vi "Movimiento_2Ejes(SubVi).vi"(2 "Cluster":T1={"Dif_1"=0.0, "Dif_2"=0.0, "Motion Resource 2"="Eje Y", "Motion Resource 1"="Eje X", "Velocidad"=0.0, "Posición_1"=0.0, "Posición_2"=0.0}) -> (0 "Done":bool)   [LabVIEW 2017]
uses:
  <vilib>/Motion/Express/_s/nimc.fb.straightLineMove.startStraightLineMove.axis.modeAbsolute.0.vi
  <vilib>/Motion/BlockNode/FB.NIMotion.xnode
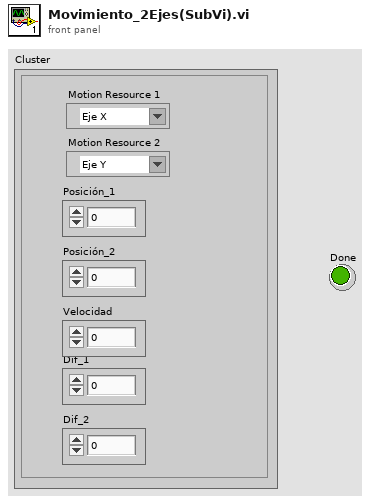
[diagram p1: front panel]
types:
  T1 = cluster{"Dif_1":dbl, "Dif_2":dbl, "Motion Resource 2":refnum<k21>, "Motion Resource 1":refnum<k21>, "Velocidad":dbl, "Posición_1":dbl, "Posición_2":dbl}
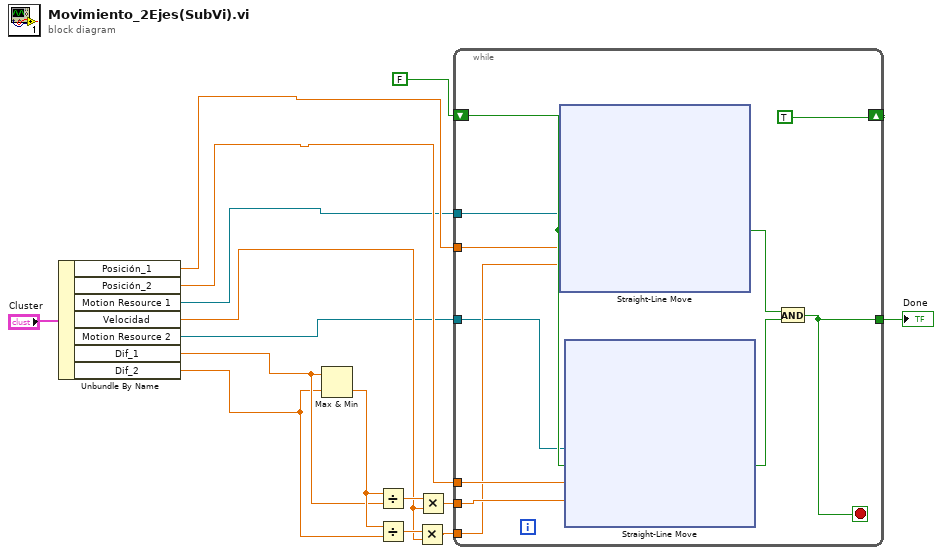
[diagram p0: block diagram]
diagram:
  n1 = Unbundle By Name("Cluster") -> ("Posición_1"=w7:dbl, "Posición_2"=w6:dbl, "Motion Resource 1"=w5:refnum<k21>, "Velocidad"=w4:dbl, "Motion Resource 2"=w3:refnum<k21>, "Dif_1"=w2:dbl, "Dif_2"=w1:dbl)
  n2 = Max & Min(x=w2, y=w1) -> (min(x,y)=w10:dbl)  [unwired: 1 out]
  n3 = Divide(x=w10, y=w2) -> (x/y=w12:dbl)
  n4 = Divide(x=w10, y=w1) -> (x/y=w11:dbl)
  n5 = Multiply(x=w11, y=w4) -> (x*y=w14:dbl)
  n6 = Multiply(x=w12, y=w4) -> (x*y=w13:dbl)
  n7 = while {
    shift-right: [TRUE] -> _
    shift-left: FALSE -> [w25]
    tunnel: [w22] -> w9
    tunnel: w7 -> [w21]
    tunnel: w6 -> [w20]
    tunnel: w14 -> [w18]
    tunnel: w13 -> [w19]
    tunnel: w5 -> [w17]
    tunnel: w3 -> [w16]
    stop <- w22 stop-if-true
    n8 = xnode "Straight-Line Move"("resource"=w17, "execute"=w25, "position"=w21, "velocity"=w18) -> ("done"=w24:bool)  [unwired: 2 in, 2 out]
    n9 = xnode "Straight-Line Move"("resource"=w16, "execute"=w25, "position"=w20, "velocity"=w19) -> ("done"=w23:bool)  [unwired: 2 in, 2 out]
    n10 = And(x=w24, y=w23) -> (x .and. y?=w22:bool)
  }
  "Done" <- w9
